vi "Add Points to Series_DBL-DBL-Name.vi"(6 "YValuesPerPoint":i32=1, 8 "error in (no error)":errorcluster, 9 "Data":cluster{"X":dbl, "Y":dbl, "Name":string}[](array[cluster])=[{"X"=0.0, "Y"=0.0, "Name"=""}, {"X"=0.0, "Y"=0.0, "Name"=""}, {"X"=0.0, "Y"=0.0, "Name"=""}, {"X"=0.0, "Y"=0.0, "Name"=""}, {"X"=0.0, "Y"=0.0, "Name"=""}, {"X"=0.0, "Y"=0.0, "Name"=""}, {"X"=0.0, "Y"=0.0, "Name"=""}, {"X"=0.0, "Y"=0.0, "Name"=""}], 10 ".NET MSChart Series":refnum<k24>) -> (0 "error out":errorcluster, 2 ".NET MSChart Series (dup)":refnum<k24>)   [LabVIEW 2014, in "XMSChart.xctl"]
uses:
  XMSChart.xctl
  System.Windows.Forms.DataVisualization
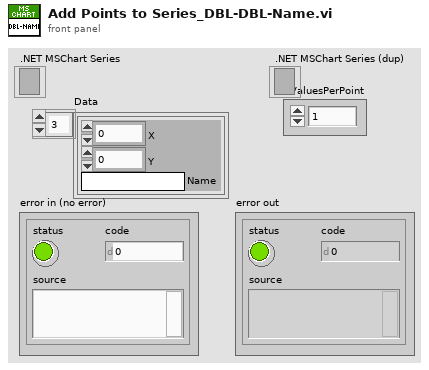
[diagram p1: front panel]
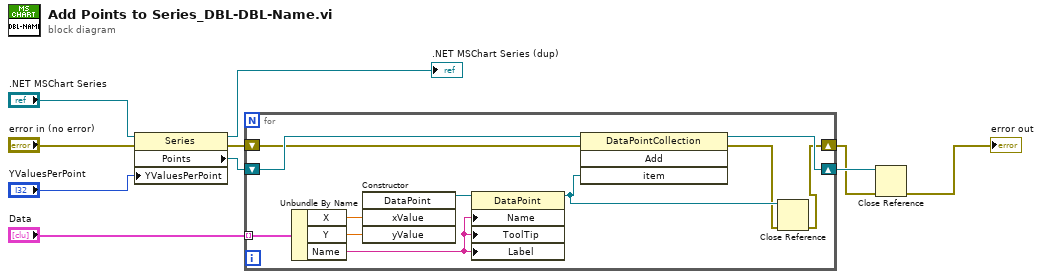
[diagram p0: block diagram]
diagram:
  n1 = property class="Series"(reference=".NET MSChart Series", error in="error in (no error)", "YValuesPerPoint"="YValuesPerPoint") -> (reference out=→".NET MSChart Series (dup)":refnum<k24>, error out=w6:errorcluster, "Points"=w7:refnum<k24>)
  n2 = for {
    tunnel: "Data" -> [w18] mode=indexing
    shift-right: [w20] -> w5
    shift-left: w7 -> [w21]
    shift-right: [w11] -> w2
    shift-left: w6 -> [w19]
    n3 = Unbundle By Name(w18) -> ("X"=w17:dbl, "Y"=w16:dbl, "Name"=w15:string)
    n4 = constructor class="DataPoint"("xValue"=w17, "yValue"=w16) -> (reference out=w14:refnum<k24>)  [unwired: 3 in, 4 out]
    n5 = property class="DataPoint"(reference=w14, "Name"=w15, "ToolTip"=w15, "Label"=w15) -> (reference out=w13:refnum<k24>)  [unwired: 1 in, 1 out]
    n6 = invoke class="DataPointCollection" method="Add"(reference=w21, error in=w19, "item"=w13) -> (reference out=w20:refnum<k24>, error out=w12:errorcluster)  [unwired: 1 in, 2 out]
    n7 = Close Reference(reference=w13, error in (no error)=w12) -> (error out=w11:errorcluster)
  }
  n8 = Close Reference(reference=w5, error in (no error)=w2) -> (error out=→"error out":errorcluster)
